vi "rest_get_latest.vi"() -> ()   [LabVIEW 2024]
uses:
  <vilib>/addons/_JKI.lib/REST Client/classes/REST Client/REST Client.lvclass
panel:
  out "value":cluster{"group_id":string, "id":i32}[](array[cluster])
  out "Response body":string
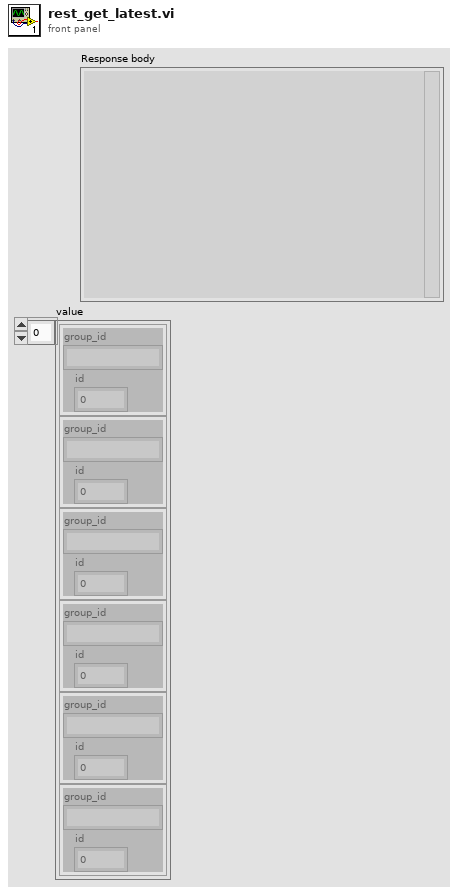
[diagram p1: front panel]
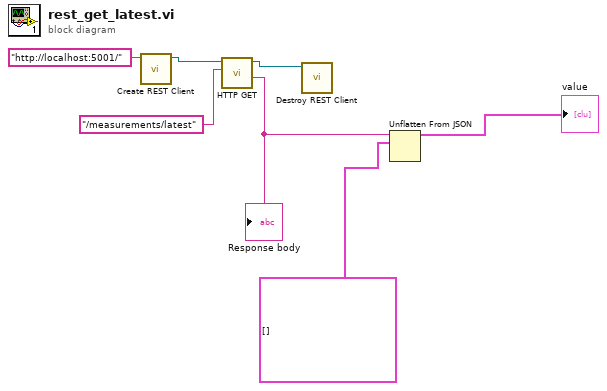
[diagram p0: block diagram]
diagram:
  n1 = call <vilib>:"Create REST Client.vi"("Base URL"="http://localhost:5001/") -> ("REST Client out"=w7:refnum<class "REST Client.lvclass">)  [unwired: 9 in, 1 out]
  n2 = call-dynamic "HTTP GET.vi"("Path"="/measurements/latest", "REST Client in"=w7) -> ("Response body"=w3:string, "REST Client out"=w6:refnum<class "REST Client.lvclass">)  [unwired: 4 in, 4 out]
  "Response body" <- w3
  n3 = call-dynamic "Destroy REST Client.vi"("REST Client in"=w6) -> ()  [unwired: 10 in, 1 out]
  n4 = Unflatten From JSON(JSON string=w3, type and defaults=cluster{"group_id":string, "id":i32}[] []) -> (value=→"value":cluster{"group_id":string, "id":i32}[])  [unwired: 5 in, 1 out]
